vi "Read Output PID Components.vi"(7 "Unit Address (1)":u8=1, 8 "error in (no error)":errorcluster, 10 "Number of PID (1)":u8=1 min=1 max=3, 11 "VISA resource name":refnum<visa-resource-name>) -> (0 "error out":errorcluster, 1 "Integral Component Output":i32, 2 "Proportional Band":i32, 3 "VISA resource name out":refnum<visa-resource-name>, 5 "Derivative Component  Output":i32)   [LabVIEW 2014, in "Eurotherm 35xx Series.lvlib"]
doc: "This VI returns Components of Output."
uses:
  <instrlib>/Eurotherm 35xx Series/Eurotherm 35xx Series.lvlib
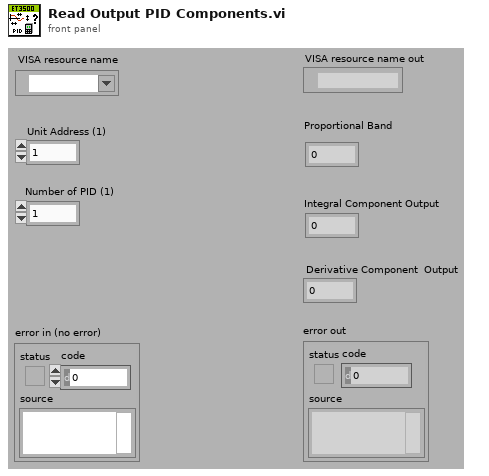
[diagram p1: front panel]
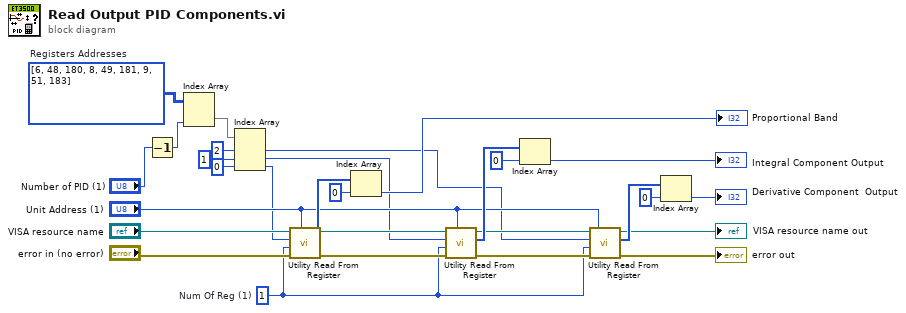
[diagram p0: block diagram]
diagram:
  w10 = u16[][] [[6, 48, 180], [8, 49, 181], [9, 51, 183]]  # Registers Addresses
  w14 = u16 1  # Num Of Reg (1)
  n1 = Decrement(x="Number of PID (1)") -> (x-1=w4:u8)
  n2 = Index Array(array=w10, index (col)=w4) -> (element=w9:u16[])  [unwired: 1 in]
  n3 = Index Array(array=w9, index #1=2 ("index"), index #2=1 ("index"), index #3=0 ("index")) -> (element #1=w1:u16, element #2=w2:u16, element #3=w3:u16)
  n4 = call <instrlib>:"Utility Read From Register.vi"("Unit Address (1)"="Unit Address (1)", "error in (no error)"="error in (no error)", "Num Of Reg (1)"=w14, "Register Address (0)"=w3, "VISA resource name"="VISA resource name") -> ("error out"=w23:errorcluster, "Data"=w27:i16[], "VISA resource name out"=w24:refnum<visa-resource-name>)  [unwired: 4 in]
  n5 = Index Array(array=w27, index=0) -> (element=→"Proportional Band":i16)
  n6 = call <instrlib>:"Utility Read From Register.vi"("Unit Address (1)"="Unit Address (1)", "error in (no error)"=w23, "Num Of Reg (1)"=w14, "Register Address (0)"=w2, "VISA resource name"=w24) -> ("error out"=w16:errorcluster, "Data"=w21:i16[], "VISA resource name out"=w17:refnum<visa-resource-name>)  [unwired: 4 in]
  n7 = Index Array(array=w21, index=0) -> (element=→"Integral Component Output":i16)
  n8 = call <instrlib>:"Utility Read From Register.vi"("Unit Address (1)"="Unit Address (1)", "error in (no error)"=w16, "Num Of Reg (1)"=w14, "Register Address (0)"=w1, "VISA resource name"=w17) -> ("error out"=→"error out":errorcluster, "Data"=w19:i16[], "VISA resource name out"=→"VISA resource name out":refnum<visa-resource-name>)  [unwired: 4 in]
  n9 = Index Array(array=w19, index=0) -> (element=→"Derivative Component  Output":i16)
